vi "ADI_IMU_ADIS16448_Open.vi"(8 "error in":errorcluster, 9 "AHRS Algorithm":enum16{"Complementary", "Madgwick"}(ring), 10 "Yaw Axis":enum16{"X", "Y", "Z"}(ring)=enum."Z", 11 "Calibrate On Open":bool=TRUE) -> (0 "error out":errorcluster, 3 "ADI IMU DevRef Out":T1={"DevStatus"={"status"=FALSE, "code"=0, "source"=""}, "Handle"=0, "SPI Bus"=enum."SPI On-Board, CS0", "Device Found"=FALSE, "Device Ready"=FALSE, "Yaw Axis"=enum."Z", "AHRS Algorithm"=enum."Complementary", "Serial"=0, "Lot ID 2"=0, "Lot ID 1"=0, "Bytes Per Sample"=0, "Calibrate On Open?"=FALSE})   [LabVIEW 2019, in "ADIS16448_IMU.lvlib"]
doc: "Initiates communication between an Analog Devices MXP IMU and the RoboRIO."
uses:
  ADIS16448_IMU.lvlib
  ADI_IMU_ADIS16448_IMUDevRef.ctl
  <vilib>/Rock Robotics/SystemInterfaces/spilib/spi_bus.ctl
  <vilib>/Rock Robotics/WPI/SPI/WPI_SPIMode.ctl
  <vilib>/Rock Robotics/SystemInterfaces/DIO/FPGA_DIOChannel.ctl
  ADI_IMU_ADIS16448_Registers.ctl
  <vilib>/Rock Robotics/SystemInterfaces/NetworkCommunication/NetComm_UsageReport_ResourceType.ctl
  <vilib>/Utility/error.llb/DialogType.ctl
  <vilib>/Rock Robotics/WPI/Counter/WPI_CounterDigitalInputToDigitalSource.vi
  ADI_IMU_ADIS16448_Loop.vi
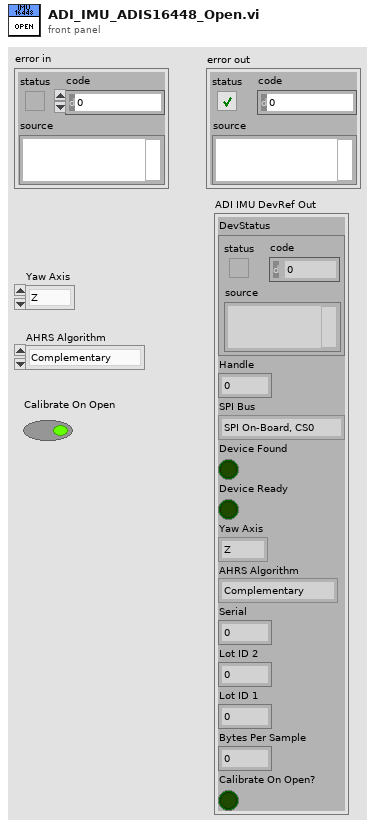
[diagram p1: front panel]
types:
  T1 = typedef "ADIS16448_IMU.lvlib/ADI_IMU_ADIS16448_IMUDevRef.ctl" = cluster{"DevStatus":errorcluster, "Handle":i32, "SPI Bus":T2, "Device Found":bool, "Device Ready":bool, "Yaw Axis":enum16{"X", "Y", "Z"}, "AHRS Algorithm":enum16{"Complementary", "Madgwick"}, "Serial":u16, "Lot ID 2":u16, "Lot ID 1":u16, "Bytes Per Sample":u16, "Calibrate On Open?":bool}
  T2 = typedef "spi_bus.ctl" = enum16{"SPI On-Board, CS0", "SPI On-Board, CS1", "SPI On-Board, CS2", "SPI On-Board, CS3", "SPI MXP", "Invalid"}
  T3 = typedef "FPGA_DIOChannel.ctl" = enum8{"DIO 0", "DIO 1", "DIO 2", "DIO 3", "DIO 4", "DIO 5", "DIO 6", "DIO 7", "DIO 8", "DIO 9", "DIO MXP 0", "DIO MXP 1", "DIO MXP 2", "DIO MXP 3", "DIO MXP 4", "DIO MXP 5", "DIO MXP 6", "DIO MXP 7", "DIO MXP 8", "DIO MXP 9", "DIO MXP 10", "DIO MXP 11", "DIO MXP 12", "DIO MXP 13", "DIO MXP 14", "DIO MXP 15", "SPI Port CS1", "SPI Port CS2", "SPI Port CS3", "SPI Port MISO", "SPI Port MOSI", "Invalid"}
  T4 = typedef "WPI_SPIMode.ctl" = enum16{"Mode 0 (Clk Idle Low,Sample on Leading)", "Mode 1 (Clk Idle Low,Sample on Trailing)", "Mode 2 (Clk Idle High,Sample on Leading)", "Mode 3 (Clk Idle High,Sample on Trailing)"}
  T5 = typedef "NetComm_UsageReport_ResourceType.ctl" = enum8{"Controller", "Module", "Language", "CANPlugin", "Accelerometer", "ADXL345", "AnalogChannel", "AnalogTrigger", "AnalogTriggerOutput", "CANJaguar", "Compressor", "Counter", "Dashboard", "DigitalInput", "DigitalOutput", "DriverStationCIO", "DriverStationEIO", "DriverStationLCD", "Encoder", "GearTooth", "Gyro", "I2C", "Framework", "Jaguar", "Joystick", "Kinect", "KinectStick", "PIDController", "Preferences", "PWM", "Relay", "RobotDrive", "SerialPort", "Servo", "Solenoid", "SPI", "Task", "Ultrasonic", "Victor", "Button", "Command", "AxisCamera", "PCVideoServer", "SmartDashboard", "Talon", "HiTechnicColorSensor", "HiTechnicAccel", "HiTechnicCompass", "SRF08", "AnalogOutput", "Victor SP", "Talon SRX", "CAN Talon SRX", "ADXL362 Accel", "ADXRS450 Gyro", "Rev SPARK", "Mindsensors SD540", "Digital Filter", "ADIS16448", "PDP", "PCM", "PigeonIMU", "Nidec Brushless", "CTRE CANifier", "CTRE TalonFX", "CTRE Future 1", "CTRE Future 2", "CTRE Future 3", "CTRE Future 4", "CTRE Future 5", "CTRE Future 6", "Linear Filter", "Xbox Controller", "USB Camera", "NavX", "Pixy", "Pixy2", "ScanseSweep", "Shuffleboard", "CAN", "Digilent DMC60", "PWM Victor SPX", "Rev SPARK MAX PWM", "Rev SPARK MAX CAN", "ADIS16470", "PIDController2", "ProfiledPIDController", "Kinematics", "Odometry", "Units", "Trapezoid Profile", "DutyCycle", "Addressable LEDs", "Fusion Venom"}
  T6 = typedef "ADIS16448_IMU.lvlib/ADI_IMU_ADIS16448_Registers.ctl" = u8
  T7 = typedef "WPI_DigitalOutputDevRef.ctl" = cluster{"DIO Channel":T3, "DevStatus":errorcluster}
  T8 = typedef "WPI_DigitalInputDevRef.ctl" = cluster{"DevStatus":errorcluster, "DIO Channel":T3}
  T9 = typedef "WPI_SPIDevRef.ctl" = cluster{"DevStatus":errorcluster, "Handle":i32, "SPI Bus":T2}
  T10 = typedef "FPGA_CounterEncoderSourceConvertionLVSourceType.ctl" = cluster{"DevStatus":errorcluster, "AnalogTriggerMode?":bool, "DigitalMode":cluster{"DIO Channel":T11}, "AnalogTriggerMode":cluster{"AnalogTriggerIndex":T12, "OutputType":T13}}
  T11 = typedef "FPGA_DIODigitalSourceChannel.ctl" = enum8{"DIO 0", "DIO 1", "DIO 2", "DIO 3", "DIO 4", "DIO 5", "DIO 6", "DIO 7", "DIO 8", "DIO 9", "DIO MXP 0", "DIO MXP 1", "DIO MXP 2", "DIO MXP 3", "DIO MXP 4", "DIO MXP 5", "DIO MXP 6", "DIO MXP 7", "DIO MXP 8", "DIO MXP 9", "DIO MXP 10", "DIO MXP 11", "DIO MXP 12", "DIO MXP 13", "DIO MXP 14", "DIO MXP 15", "SPI Port CS1", "SPI Port CS2", "SPI Port CS3", "SPI Port MISO", "SPI Port MOSI", "Disabled"}
  T12 = typedef "FPGA_AnalogTriggerIndex.ctl" = enum8{"Trig 0", "Trig 1", "Trig 2", "Trig 3", "Trig 4", "Trig 5", "Trig 6", "Trig 7", "Invalid"}
  T13 = typedef "FPGA_AnalogTriggerOutType.ctl" = enum16{"InWindow", "TriggerState", "Rising", "Falling"}
  T14 = typedef "DialogType.ctl" = u16
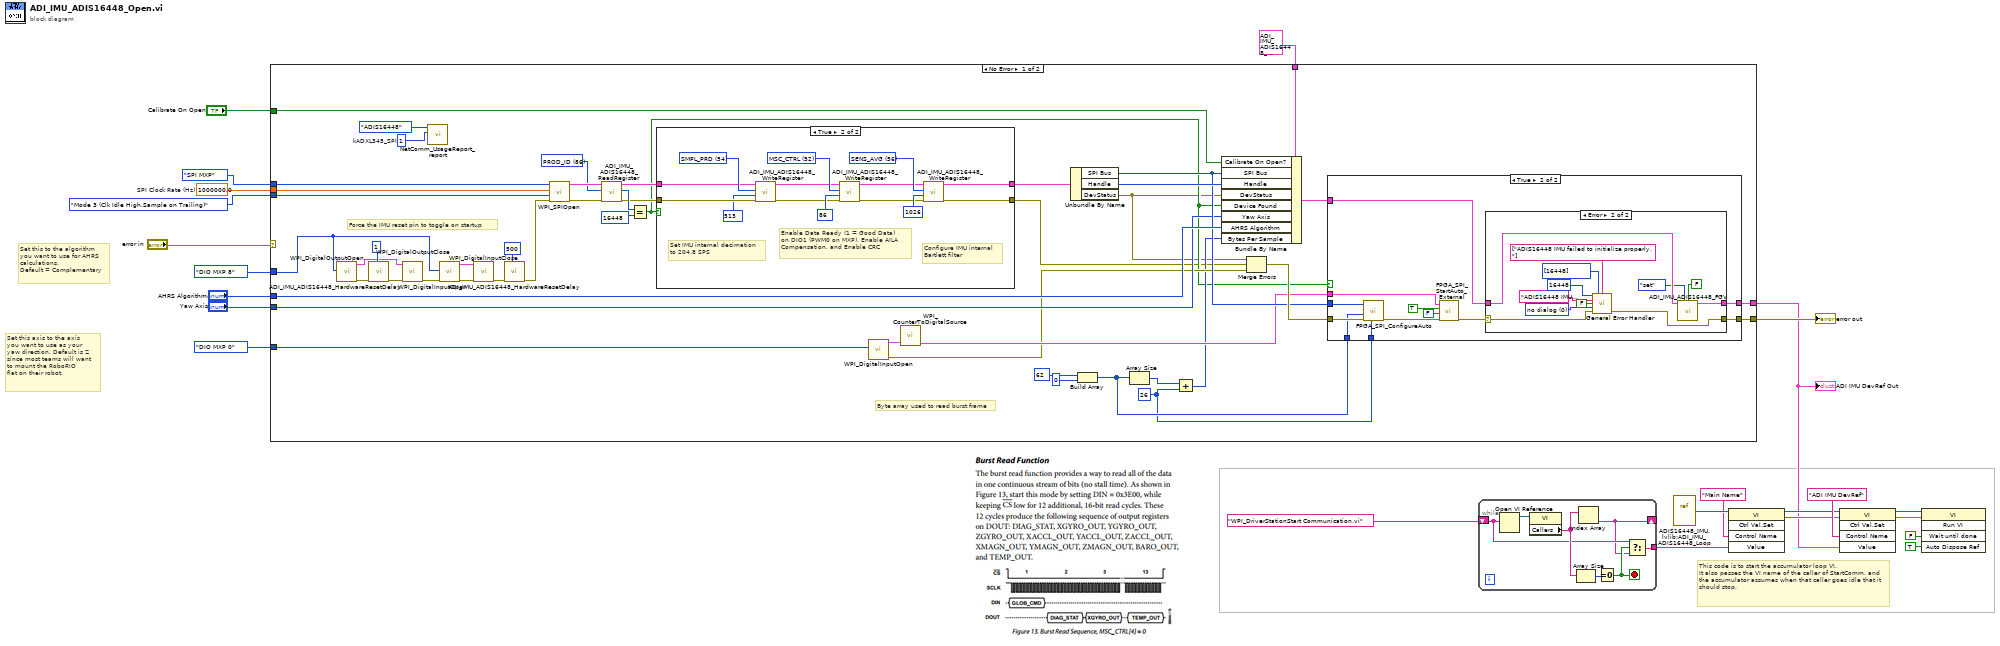
[diagram p0: block diagram]
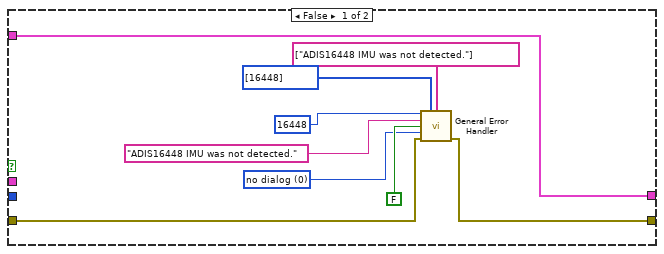
[diagram p2: hidden frame]
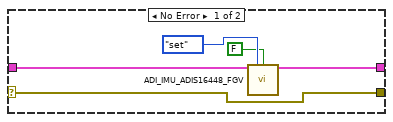
[diagram p3: hidden frame]
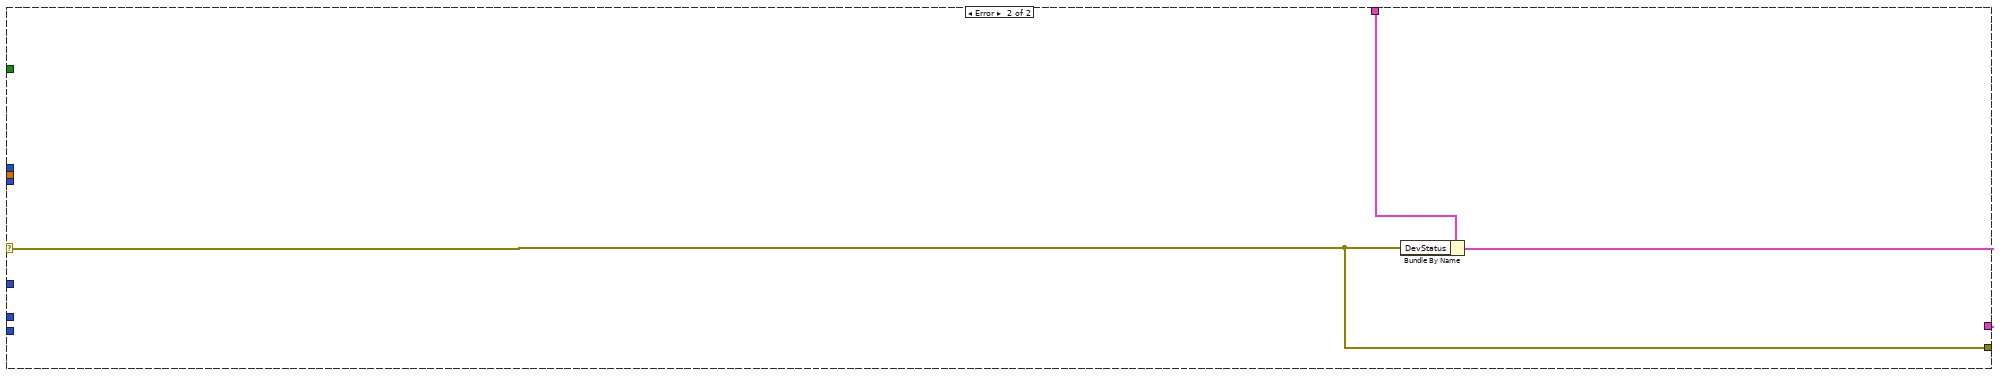
[diagram p5: hidden frame]
diagram:
  w23 = 1000000.0  # SPI Clock Rate (Hz)
  # "This code is to start the accumulator loop VI.\nIt also passes the VI name of the caller of StartComm, and the accumulator assumes when that caller goes idle that it should stop."
  # "Set this to the algorithm\nyou want to use for AHRS\ncalculations. \nDefault = Complementary"
  # "Set this axis to the axis\nyou want to use as your\nyaw direction. Default is Z\nsince most teams will want \nto mount the RoboRIO\nflat on their robot."
  n1 = case shown="No Error" "error in" {
    selector: "error in" -> [_ w126]
    tunnel: w23 -> [w70 _]
    tunnel: WPI_SPIMode."Mode 3 (Clk Idle High,Sample on Trailing)" ("Mode (3)") -> [w69 _]
    tunnel: spi_bus."SPI MXP" ("SPI Chip Select") -> [w68 _]
    tunnel: FPGA_DIOChannel."DIO MXP 0" ("DIO Channel") -> [w51 _]
    tunnel: "Yaw Axis" -> [w48 _]
    tunnel: "AHRS Algorithm" -> [w67 _]
    tunnel: FPGA_DIOChannel."DIO MXP 8" ("DIO Channel") -> [w66 _]
    tunnel: "Calibrate On Open" -> [w32 _]
    tunnel: T1 {"DevStatus"={"status"=FALSE, "code"=0, "source"=""}, "Handle"=0, "SPI Bus"=enum."SPI On-Board, CS0", "Device Found"=FALSE, "Device Ready"=FALSE, "Yaw Axis"=enum."Z", "AHRS Algorithm"=enum."Complementary", "Serial"=0, "Lot ID 2"=0, "Lot ID 1"=0, "Bytes Per Sample"=0, "Calibrate On Open?"=FALSE} ("SimpleGyroDevRef 2") -> [w47 w127]
    tunnel: [w46 w126] -> w2
    tunnel: [w24 w125] -> w1
    frame No Error {
      w29 = 26 ("dimension size")
      w63 = u8 1  # kADXL345_SPI
      w59 = T6 86 items=["GLOB_CMD"=62, "SEQ_CNT"=58, "SMPL_PRD"=54, "SENS_AVG"=56, "MSC_CTRL"=52, "ERROR_FLAGS"=60, "TEMP"=44, "BARO"=40, "Z_MAG"=36, "Y_MAG"=32, "X_MAG"=28, "Z_ACCEL"=24, "Y_ACCEL"=20, "X_ACCEL"=16, "Z_GYRO"=12, "Y_GYRO"=8, "X_GYRO"=4, "PROD_ID"=86, "LOT_ID2"=84, "LOT_ID1"=82, "SERIAL_NUM"=88] ("ADIS16448 Register")
      # "Byte array used to read burst frame"
      # "Force the IMU reset pin to toggle on startup"
      n2 = call <vilib>:"WPI_DigitalOutputOpen.vi"("DIO Channel"=w66) -> ("error out"=w43:errorcluster, "DigitalOutputDevRef"=w37:T7)  [unwired: 9 in]
      n3 = call "ADI_IMU_ADIS16448_HardwareResetDelay.vi"("Delay (ms)"=u32 1, "error in"=w43) -> ("error out"=w44:errorcluster)  [unwired: 9 in]
      n4 = call <vilib>:"WPI_DigitalOutputClose.vi"("error in (no error)"=w44, "DigitalOutputDevRef"=w37) -> ("error out"=w42:errorcluster)  [unwired: 9 in]
      n5 = call <vilib>:"NetComm_UsageReport_report.vi"("Instance Number"=w63, "Resource Type"=NetComm_UsageReport_ResourceType."ADIS16448") -> ()  [unwired: 10 in]
      n6 = call <vilib>:"WPI_DigitalInputOpen.vi"("error in (no error)"=w42, "DIO Channel"=w66) -> ("error out"=w41:errorcluster, "DigitalInputDevRef"=w40:T8)  [unwired: 8 in]
      n7 = call <vilib>:"WPI_DigitalInputClose.vi"("error in (no error)"=w41, "DigitalInputDevRef"=w40) -> ("error out"=w39:errorcluster)  [unwired: 9 in]
      n8 = call "ADI_IMU_ADIS16448_HardwareResetDelay.vi"("Delay (ms)"=u32 500, "error in"=w39) -> ("error out"=w64:errorcluster)  [unwired: 9 in]
      n9 = call <vilib>:"WPI_SPIOpen.vi"("error in"=w64, "Mode (3)"=w69, "Clock Rate (Hz)"=w70, "SPI Bus"=w68) -> ("error out"=w60:errorcluster, "SPIDevRef"=w61:T9)  [unwired: 6 in]
      n10 = call "ADI_IMU_ADIS16448_ReadRegister.vi"("error in (no error)"=w60, "ADIS16448 Register"=w59, "SPIDevRef in"=w61) -> ("error out"=w55:errorcluster, "Register Value"=w58:u16, "SPIDevRef out"=w56:T9)  [unwired: 6 in]
      n11 = Equal?(x=w58, y=u16 16448) -> (x = y?=w28:bool)
      n12 = case shown="True" w28 {
        tunnel: [w110 w112] -> w54
        tunnel: [w109 w111] -> w26
        tunnel: w56 -> [w110 w115]
        tunnel: w55 -> [w109 w114]
        frame False {
        }
        frame True {
          w120 = T6 56 items=["GLOB_CMD"=62, "SEQ_CNT"=58, "SMPL_PRD"=54, "SENS_AVG"=56, "MSC_CTRL"=52, "ERROR_FLAGS"=60, "TEMP"=44, "BARO"=40, "Z_MAG"=36, "Y_MAG"=32, "X_MAG"=28, "Z_ACCEL"=24, "Y_ACCEL"=20, "X_ACCEL"=16, "Z_GYRO"=12, "Y_GYRO"=8, "X_GYRO"=4, "PROD_ID"=86, "LOT_ID2"=84, "LOT_ID1"=82, "SERIAL_NUM"=88] ("ADIS16448 Register")
          w121 = T6 52 items=["GLOB_CMD"=62, "SEQ_CNT"=58, "SMPL_PRD"=54, "SENS_AVG"=56, "MSC_CTRL"=52, "ERROR_FLAGS"=60, "TEMP"=44, "BARO"=40, "Z_MAG"=36, "Y_MAG"=32, "X_MAG"=28, "Z_ACCEL"=24, "Y_ACCEL"=20, "X_ACCEL"=16, "Z_GYRO"=12, "Y_GYRO"=8, "X_GYRO"=4, "PROD_ID"=86, "LOT_ID2"=84, "LOT_ID1"=82, "SERIAL_NUM"=88] ("ADIS16448 Register")
          w122 = T6 54 items=["GLOB_CMD"=62, "SEQ_CNT"=58, "SMPL_PRD"=54, "SENS_AVG"=56, "MSC_CTRL"=52, "ERROR_FLAGS"=60, "TEMP"=44, "BARO"=40, "Z_MAG"=36, "Y_MAG"=32, "X_MAG"=28, "Z_ACCEL"=24, "Y_ACCEL"=20, "X_ACCEL"=16, "Z_GYRO"=12, "Y_GYRO"=8, "X_GYRO"=4, "PROD_ID"=86, "LOT_ID2"=84, "LOT_ID1"=82, "SERIAL_NUM"=88] ("ADIS16448 Register")
          # "Configure IMU internal\nBartlett filter"
          # "Enable Data Ready (1 = Good Data) \non DIO1 (PWM0 on MXP), Enable AILA\nCompensation, and Enable CRC"
          # "Set IMU internal decimation\nto 204.8 SPS"
          n13 = call "ADI_IMU_ADIS16448_WriteRegister.vi"("error in (no error)"=w114, "Data"=u16 513, "ADIS16448 Register"=w122, "SPIDevRef in"=w115) -> ("error out"=w118:errorcluster, "SPIDevRef out"=w119:T9)  [unwired: 6 in]
          n14 = call "ADI_IMU_ADIS16448_WriteRegister.vi"("error in (no error)"=w118, "Data"=u16 86, "ADIS16448 Register"=w121, "SPIDevRef in"=w119) -> ("error out"=w116:errorcluster, "SPIDevRef out"=w117:T9)  [unwired: 6 in]
          n15 = call "ADI_IMU_ADIS16448_WriteRegister.vi"("error in (no error)"=w116, "Data"=u16 1026, "ADIS16448 Register"=w120, "SPIDevRef in"=w117) -> ("error out"=w111:errorcluster, "SPIDevRef out"=w112:T9)  [unwired: 6 in]
        }
      }
      n16 = call <vilib>:"WPI_DigitalInputOpen.vi"("DIO Channel"=w51) -> ("error out"=w36:errorcluster, "DigitalInputDevRef"=w50:T8)  [unwired: 9 in]
      n17 = call-poly <vilib>:"WPI_CounterToDigitalSource.vi"("DigitalInputDevRef"=w50) -> ("Digital Source"=w49:T10)  [unwired: 6 in]
      n18 = Unbundle By Name(w54) -> ("SPI Bus"=w52:T2, "Handle"=w65:i32, "DevStatus"=w27:errorcluster)
      n19 = Build Array(u8 62 ("hi"), u8 0 ("element")) -> (w33:u8[])
      n20 = Array Size(array=w33) -> (size(s)=w31:i32)
      n21 = Add(x=w31, y=w29) -> (x+y=w30:i32)
      n22 = Bundle By Name(cluster=w47, "Calibrate On Open?"=w32, "SPI Bus"=w52, "Handle"=w65, "DevStatus"=w27, "Device Found"=w28, "Yaw Axis"=w48, "AHRS Algorithm"=w67, "Bytes Per Sample"=w30) -> (w25:T1)
      n23 = Merge Errors(w27, w26, w36) -> (w53:errorcluster)
      n24 = case shown="True" w28 {
        tunnel: w53 -> [w72 w91]
        tunnel: w52 -> [_ w90]
        tunnel: w33 -> [_ w85]
        tunnel: w49 -> [_ w86]
        tunnel: [w73 w82] -> w46
        tunnel: w29 -> [_ w84]
        tunnel: w25 -> [w71 w81]
        tunnel: [w71 w80] -> w24
        frame False {
          w76 = T14 0 items=["no dialog", "OK message", "continue or stop message", "OK message + warnings", "continue/stop + warnings"] ("type of dialog (OK msg:1)")
          n25 = call <vilib>:"General Error Handler.vi"("[error code] (0)"=16448, "[user-defined codes]"=i32[] [16448], "[user-defined descriptions]"=string[] ["ADIS16448 IMU was not detected."], "[error source] (\" \")"="ADIS16448 IMU was not detected." ("[error source] (\" \")"), "search ni.com link visible?(T)"=FALSE, "type of dialog (OK msg:1)"=w76, "error in (no error)"=w72) -> ("error out"=w73:errorcluster)  [unwired: 4 in, 4 out]
        }
        frame True {
          n26 = call <vilib>:"FPGA_SPI_ConfigureAuto.vi"("SPI Auto Zero Byte Count"=w84, "error in"=w91, "SPI Auto TX Byte Array"=w85, "SPI Bus"=w90) -> ("error out"=w89:errorcluster)  [unwired: 7 in]
          n27 = call <vilib>:"FPGA_SPI_StartAuto_External.vi"("error in (no error)"=w89, "Falling Edge"=FALSE, "Rising Edge"=TRUE, "Source"=w86) -> ("error out"=w83:errorcluster)  [unwired: 7 in]
          n28 = case shown="Error" w83 {
            selector: w83 -> [w92 w102]
            tunnel: w81 -> [w93 w100]
            tunnel: [w92 w97] -> w82
            tunnel: [w94 w101] -> w80
            frame No Error {
              n29 = call "ADI_IMU_ADIS16448_FGV.vi"("ADI IMU DevRef"=w93, "Operation"=enum16{"set", "get", "set reset"}."set", "Sensor Ready?"=FALSE) -> ("ADI IMU DevRef Out"=w94:T1)  [unwired: 6 in, 6 out]
            }
            frame Error {
              w105 = T14 0 items=["no dialog", "OK message", "continue or stop message", "OK message + warnings", "continue/stop + warnings"] ("type of dialog (OK msg:1)")
              n30 = call <vilib>:"General Error Handler.vi"("[error code] (0)"=16448, "[user-defined codes]"=i32[] [16448], "[user-defined descriptions]"=string[] ["ADIS16448 IMU failed to initialize properly."], "[error source] (\" \")"="ADIS16448 IMU failed to initialize properly." ("[error source] (\" \")"), "search ni.com link visible?(T)"=FALSE, "type of dialog (OK msg:1)"=w105, "error in (no error)"=w102) -> ("error out"=w97:errorcluster)  [unwired: 4 in, 4 out]
              n31 = call "ADI_IMU_ADIS16448_FGV.vi"("ADI IMU DevRef"=w100, "Operation"=enum16{"set", "get", "set reset"}."set", "Sensor Ready?"=FALSE) -> ("ADI IMU DevRef Out"=w101:T1)  [unwired: 6 in, 6 out]
            }
          }
        }
      }
    }
    frame Error {
      n32 = Bundle By Name(cluster=w127, "DevStatus"=w126) -> (w125:T1)
    }
  }
  "error out" <- w2
  "ADI IMU DevRef Out" <- w1
  n33 = while {
    shift-right: [w129] -> _
    shift-left: "WPI_DriverStationStart Communication.vi" -> [w130]
    tunnel: [w128] -> w7
    stop <- w131 stop-if-true
    n34 = Open VI Reference(vi path=w130) -> (vi reference=w134:refnum<vi>)  [unwired: 1 in, 5 out]
    n35 = property class="VI"(reference=w134) -> ("Callers"=w132:string[])  [unwired: 1 in, 2 out]
    n36 = Array Size(array=w132) -> (size(s)=w133:i32)
    n37 = Index Array(array=w132) -> (element=w129:string)  [unwired: 1 in]
    n38 = Equal To 0?(x=w133) -> (x = 0?=w131:bool)
    n39 = Select(t=w130, s=w131, f=w129) -> (s? t:f=w128:string)
  }
  n40 = vi-ref "ADIS16448_IMU.lvlib:ADI_IMU_ADIS16448_Loop.vi"() -> (w9:refnum<vi>)
  n41 = invoke class="VI" method="Ctrl Val.Set"(reference=w9, "Control Name"="Main Name", "Value"=w7) -> (reference out=w6:refnum<vi>, error out=w11:errorcluster)  [unwired: 2 in, 3 out]
  n42 = invoke class="VI" method="Ctrl Val.Set"(reference=w6, error in=w11, "Control Name"="ADI IMU DevRef", "Value"=w1) -> (reference out=w16:refnum<vi>, error out=w12:errorcluster)  [unwired: 1 in, 3 out]
  n43 = invoke class="VI" method="Run VI"(reference=w16, error in=w12, "Wait until done"=FALSE ("Wait Until Done"), "Auto Dispose Ref"=TRUE ("Auto Dispose Reference")) -> ()  [unwired: 1 in, 5 out]
